vi "Ismatec 78001 Test Program.vi"() -> ()   [LabVIEW 2018, in "Ismatec 4308.lvlib"]
uses:
  Ismatec 4308.lvlib
  Ismatec 78001.ctl
  Ismatec 78001 Global.ctl
  Ismatec 78001 Global Element.ctl
panel:
  out "error out 4":errorcluster
  out "No Pump Connected":bool=TRUE
  out "Initialized":bool
  out "RPM":dbl
  out "Ismatech 3 Channel Settings Out":T1={"VISA resource name"="", "Pump Number"=1, "Channel Number"=0, "Simulated?"=TRUE, "Reverse?"=FALSE} {"Channel Number" min=0 max=3; "Pump Number" min=1 max=9}
  in  "Ismatech 3 Channel Settings In":T1={"VISA resource name"="COM5", "Pump Number"=6, "Channel Number"=1, "Simulated?"=FALSE, "Reverse?"=FALSE} {"Channel Number" min=0 max=3; "Pump Number" min=1 max=9}
  out "error out":errorcluster
  in  "error in (no error)":errorcluster
  in  "Speed (%)":dbl
  in  "Pause":bool
  out "Connection Error":bool
  out "Pump On?":enum16{"Off", "On", "Not Initialized"}(ring)
  out "Connection Error 2":bool
  in  "stop":bool
  out "error out 2":errorcluster
  out "error out 3":errorcluster
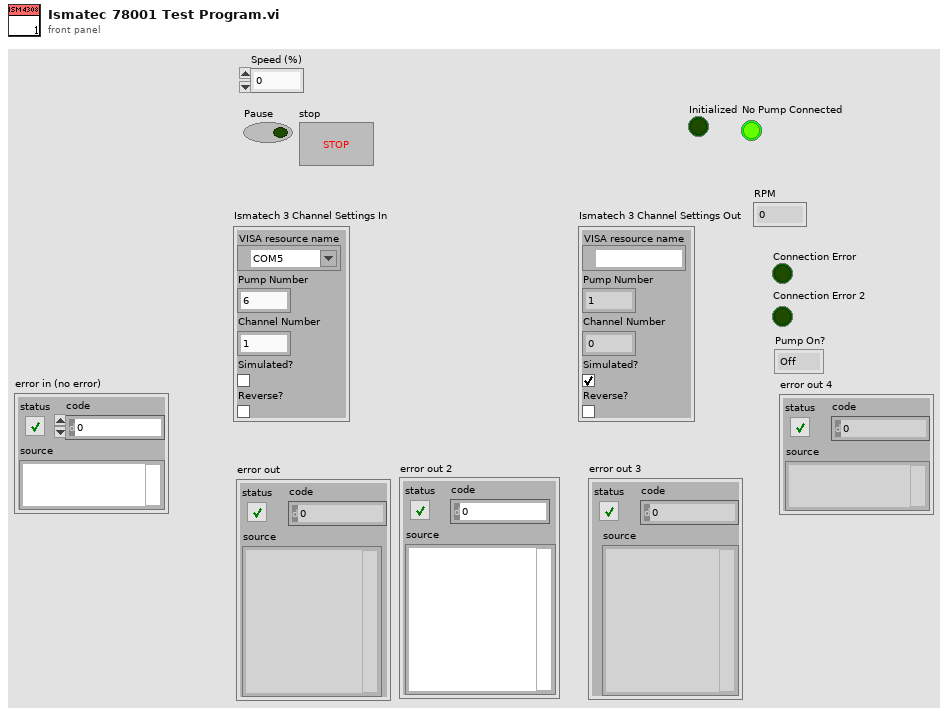
[diagram p1: front panel]
types:
  T1 = typedef "Ismatec 4308.lvlib/Ismatec 78001.ctl" = cluster{"VISA resource name":refnum<visa-resource-name>, "Pump Number":i16, "Channel Number":i16, "Simulated?":bool, "Reverse?":bool}
  T2 = typedef "Ismatec 4308.lvlib/Ismatec 78001 Global.ctl" = T3[]
  T3 = typedef "Ismatec 4308.lvlib/Ismatec 78001 Global Element.ctl" = cluster{"Busy":bool, "ChannelCnt":dbl, "Initialized":bool}
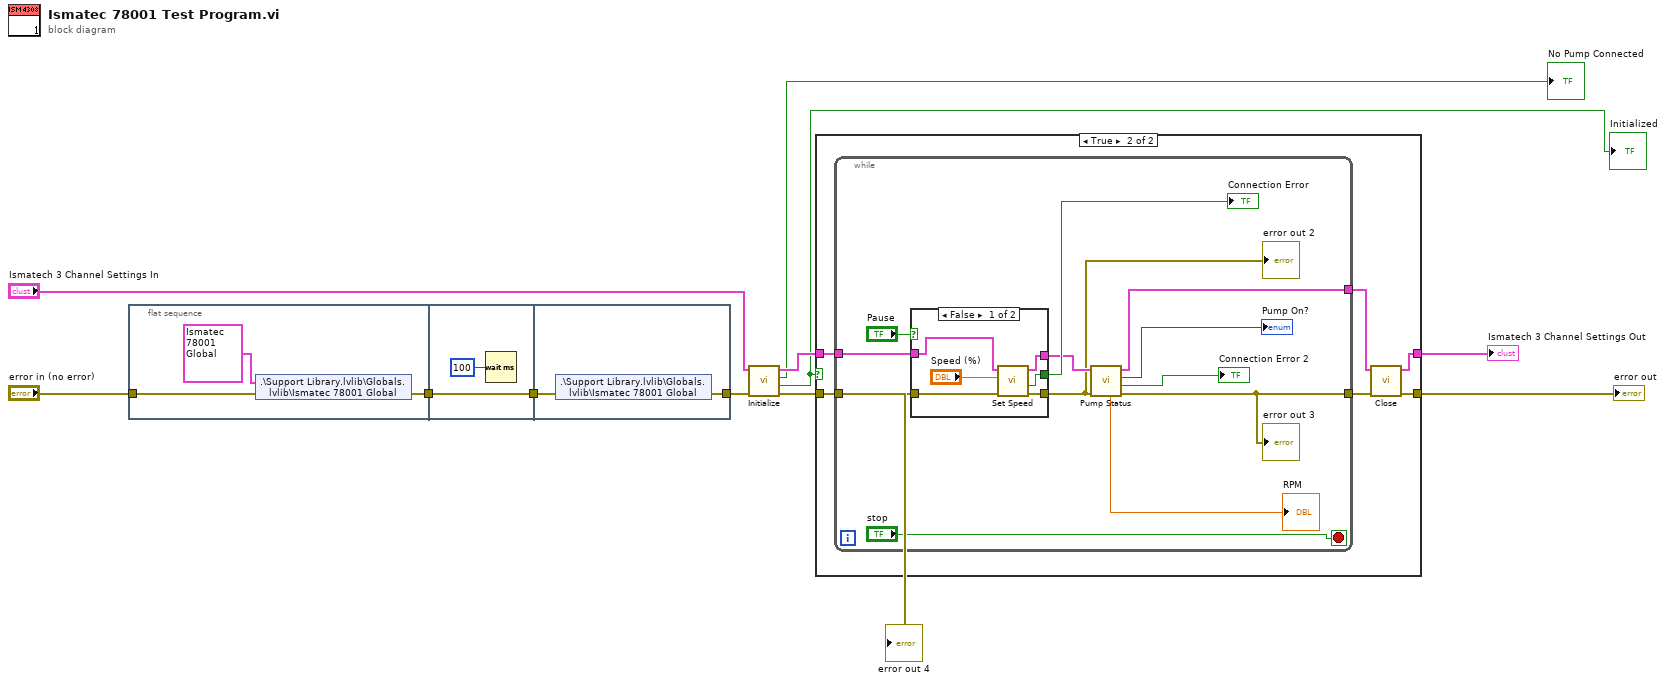
[diagram p0: block diagram]
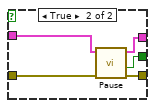
[diagram p3: hidden frame]
diagram:
  n1 = flat-sequence {
    tunnel: [w14] -> w11
    tunnel: "error in (no error)" -> [w13]
    tunnel: w11 -> [w16]
    tunnel: [w16] -> w10
    tunnel: w10 -> [w17]
    tunnel: [w18] -> w6
    frame #0 {
      n2 = shared-variable ".\\Support Library.lvlib\\Globals.lvlib\\Ismatec 78001 Global"(T2 [{"Busy"=FALSE, "ChannelCnt"=0.0, "Initialized"=FALSE}, {"Busy"=FALSE, "ChannelCnt"=0.0, "Initialized"=FALSE}, {"Busy"=FALSE, "ChannelCnt"=0.0, "Initialized"=FALSE}, {"Busy"=FALSE, "ChannelCnt"=0.0, "Initialized"=FALSE}, {"Busy"=FALSE, "ChannelCnt"=0.0, "Initialized"=FALSE}, {"Busy"=FALSE, "ChannelCnt"=0.0, "Initialized"=FALSE}, {"Busy"=FALSE, "ChannelCnt"=0.0, "Initialized"=FALSE}, {"Busy"=FALSE, "ChannelCnt"=0.0, "Initialized"=FALSE}, {"Busy"=FALSE, "ChannelCnt"=0.0, "Initialized"=FALSE}, {"Busy"=FALSE, "ChannelCnt"=0.0, "Initialized"=FALSE}, {"Busy"=FALSE, "ChannelCnt"=0.0, "Initialized"=FALSE}, {"Busy"=FALSE, "ChannelCnt"=0.0, "Initialized"=FALSE}, {"Busy"=FALSE, "ChannelCnt"=0.0, "Initialized"=FALSE}, {"Busy"=FALSE, "ChannelCnt"=0.0, "Initialized"=FALSE}, {"Busy"=FALSE, "ChannelCnt"=0.0, "Initialized"=FALSE}, {"Busy"=FALSE, "ChannelCnt"=0.0, "Initialized"=FALSE}, {"Busy"=FALSE, "ChannelCnt"=0.0, "Initialized"=FALSE}, {"Busy"=FALSE, "ChannelCnt"=0.0, "Initialized"=FALSE}, {"Busy"=FALSE, "ChannelCnt"=0.0, "Initialized"=FALSE}, {"Busy"=FALSE, "ChannelCnt"=0.0, "Initialized"=FALSE}, {"Busy"=FALSE, "ChannelCnt"=0.0, "Initialized"=FALSE}] ("Array"), error in=w13) -> (error out=w14:errorcluster)
    }
    frame #1 {
      n3 = Wait (ms)(milliseconds to wait=u32 100) -> ()  [unwired: 1 out]
    }
    frame #2 {
      n4 = shared-variable ".\\Support Library.lvlib\\Globals.lvlib\\Ismatec 78001 Global"(error in=w17) -> (error out=w18:errorcluster)  [unwired: 1 out]
    }
  }
  n5 = call "Initialize.vi"("error in (no error)"=w6, "Ismatech 3 Channel Settings In"="Ismatech 3 Channel Settings In") -> ("error out"=w7:errorcluster, "Initialized"=w3:bool, "No Pump Connected"=→"No Pump Connected":bool, "Ismatech 3 Channel Settings Out"=w8:T1)  [unwired: 6 in]
  "Initialized" <- w3
  "error out 4" <- w7
  n6 = case shown="True" w3 {
    tunnel: w8 -> [w19 w26]
    tunnel: w7 -> [w20 w25]
    tunnel: [w20 w22] -> w2
    tunnel: [w19 w21] -> w1
    frame False {
    }
    frame True {
      n7 = while {
        tunnel: w26 -> [w37]
        tunnel: w25 -> [w36]
        tunnel: [w31] -> w23
        tunnel: [w28] -> w24
        stop <- "stop" stop-if-true
        n8 = case shown="False" "Pause" {
          tunnel: w37 -> [w43 w45]
          tunnel: w36 -> [w42 w46]
          tunnel: [w41 w48] -> w33
          tunnel: [w39 w47] -> w32
          tunnel: [w40 w49] -> w35
          frame False {
            n9 = call "Set Speed.vi"("error in (no error)"=w42, "Speed (%)"="Speed (%)", "Ismatech 3 Channel Settings In"=w43) -> ("error out"=w39:errorcluster, "Connection Error"=w40:bool, "Ismatech 3 Channel Settings Out"=w41:T1)  [unwired: 5 in, 1 out]
          }
          frame True {
            n10 = call "Pause.vi"("error in (no error)"=w46, "Ismatech 3 Channel Settings In"=w45) -> ("error out"=w47:errorcluster, "Connection Error"=w49:bool, "Ismatech 3 Channel Settings Out"=w48:T1)  [unwired: 6 in, 1 out]
          }
        }
        "Connection Error" <- w35
        "error out 2" <- w32
        n11 = call "Pump Status.vi"("error in (no error)"=w32, "Ismatech 3 Channel Settings In"=w33) -> ("error out"=w28:errorcluster, "Connection Error"=→"Connection Error 2":bool, "Pump On?"=→"Pump On?":enum16{"Off", "On", "Not Initialized"}, "Ismatech 3 Channel Settings Out"=w31:T1, "RPM"=→"RPM":dbl)  [unwired: 5 in]
        "error out 3" <- w28
      }
      n12 = call "Close.vi"("error in (no error)"=w24, "Ismatech 3 Channel Settings In"=w23) -> ("error out"=w22:errorcluster, "Ismatech 3 Channel Settings Out"=w21:T1)  [unwired: 7 in, 1 out]
    }
  }
  "error out" <- w2
  "Ismatech 3 Channel Settings Out" <- w1
